vi "伏安特性.vi"() -> ()   [LabVIEW 2014]
uses:
  <vilib>/Analysis/NI_AALPro.lvlib
panel:
  in  "开关":bool
  out "数据":dbl[][](array[numeric])
  out "待测电阻值":dbl
  in  "时间间隔":dbl[unit]
  in  "标准电阻":dbl
  in  "测量数据点数":dbl
  in  "输出电压步长":dbl[unit]
  out "电阻的伏安曲线图":cluster{"Y":dbl[], "Y":dbl[]}[](graph)
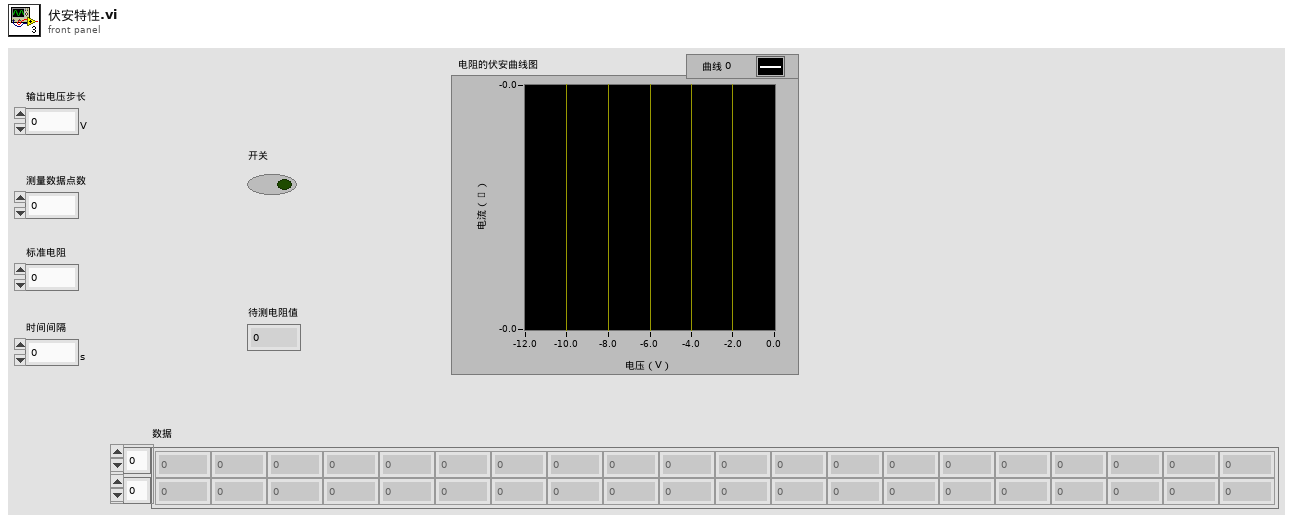
[diagram p1: front panel]
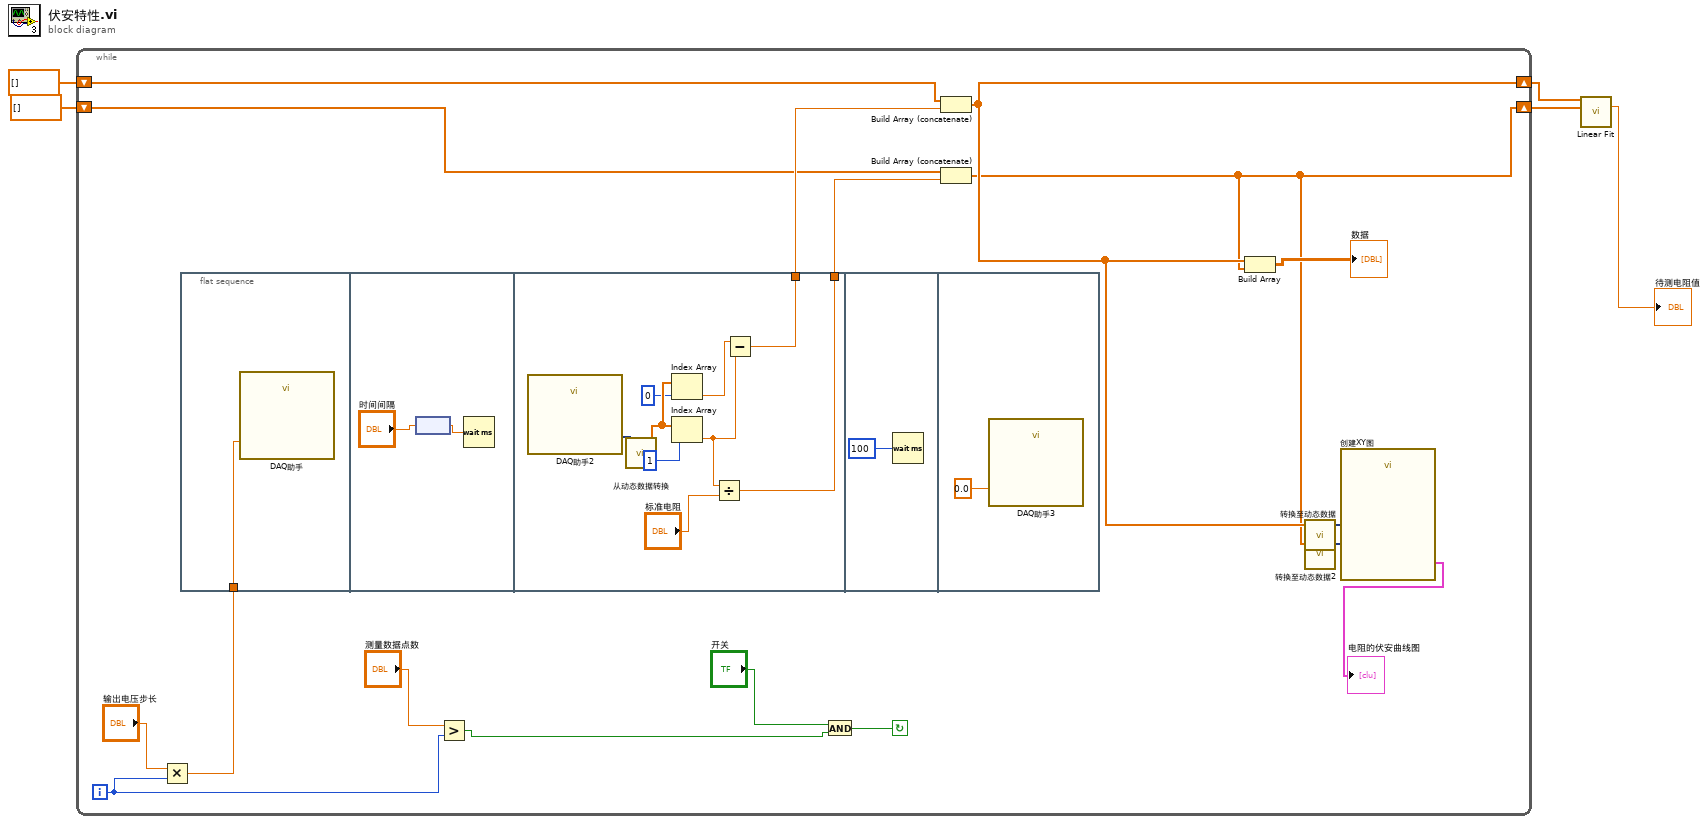
[diagram p0: block diagram]
diagram:
  n1 = while {
    shift-right: [w9] -> w3
    shift-left: dbl[] [] -> [w14]
    shift-right: [w7] -> w2
    shift-left: dbl[] [] -> [w12]
    i -> [w18]
    stop <- w15 continue-if-true
    n2 = Multiply(x="输出电压步长", y=w18) -> (x*y=w20:dbl[unit])
    n3 = flat-sequence {
      tunnel: w20 -> [w23]
      tunnel: [w27] -> w13
      tunnel: [w26] -> w11
      frame #0 {
        n4 = call "DAQ助手"("data"=w23) -> ()  [unwired: 17 in, 2 out]
      }
      frame #1 {
        n5 = node("时间间隔") -> (w25:dbl)
        n6 = Wait (ms)(milliseconds to wait=w25) -> ()  [unwired: 1 out]
      }
      frame #2 {
        n7 = call "DAQ助手2"() -> ("data"=w34:dynamicdata)  [unwired: 17 in, 2 out]
        n8 = call "从动态数据转换"("Dynamic Data Type"=w34) -> ("Array"=w33:dbl[])  [unwired: 3 in]
        n9 = Index Array(array=w33, index=0 ("索引")) -> (element=w30:dbl)
        n10 = Index Array(array=w33, index=1 ("索引")) -> (element=w29:dbl)
        n11 = Divide(x=w29, y="标准电阻") -> (x/y=w26:dbl)
        n12 = Subtract(x=w30, y=w29) -> (x-y=w27:dbl)
      }
      frame #3 {
        n13 = Wait (ms)(milliseconds to wait=u32 100 ("等待时间（毫秒）")) -> ()  [unwired: 1 out]
      }
      frame #4 {
        n14 = call "DAQ助手3"("data"=0.0 ("数据")) -> ()  [unwired: 17 in, 2 out]
      }
    }
    n15 = Greater?(x="测量数据点数", y=w18) -> (0:w17:bool)
    n16 = And(x="开关", y=w17) -> (x .and. y?=w15:bool)
    n17 = Build Array (concatenate)(w14, w13) -> (w9:dbl[])
    n18 = Build Array (concatenate)(w12, w11) -> (w7:dbl[])
    n19 = Build Array(w9, w7) -> (→"数据":dbl[][])
    n20 = call "转换至动态数据"("Array"=w9) -> ("Dynamic Data Type"=w8:dynamicdata)  [unwired: 3 in]
    n21 = call "转换至动态数据2"("Array"=w7) -> ("Dynamic Data Type"=w6:dynamicdata)  [unwired: 3 in]
    n22 = call "创建XY图"("Y Input"=w6, "X Input"=w8) -> ("XY Graph"=→"电阻的伏安曲线图":cluster{"X":dbl[], "Y":dbl[]}[])  [unwired: 8 in, 1 out]
  }
  n23 = call <vilib>:"Linear Fit.vi"("Y"=w3, "X"=w2) -> ("slope"=→"待测电阻值":dbl)  [unwired: 9 in, 4 out]
